vi "DtOLGetBoardNames.vi"(8 "error in (no error)":errorcluster, 10 "Select Board":u32) -> (0 "error out":errorcluster, 1 "Board Name":string, 2 "Number of boards":u32)   [LabVIEW 2022 SP3]
uses:
  DtLvLink.lvlib
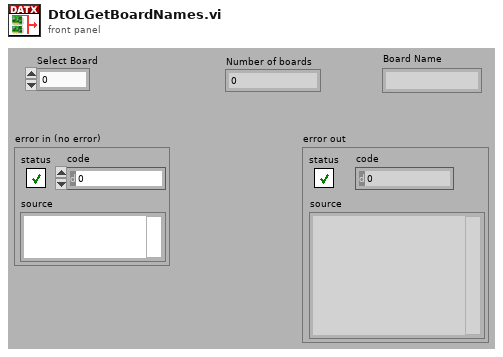
[diagram p1: front panel]
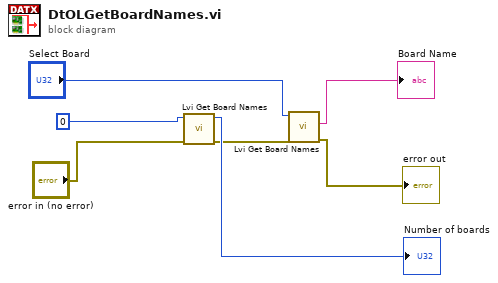
[diagram p0: block diagram]
diagram:
  n1 = call "Lvi Get Board Names.vi"("error in (no error)"="error in (no error)", "BoardNumber"=u32 0) -> ("error out"=w4:errorcluster, "NumBoardsFound"=→"Number of boards":u32)  [unwired: 6 in, 2 out]
  n2 = call "Lvi Get Board Names.vi"("error in (no error)"=w4, "BoardNumber"="Select Board") -> ("error out"=→"error out":errorcluster, "BoardName"=→"Board Name":string)  [unwired: 6 in, 2 out]
